vi "RTTrapTest-07-06-2017.vi"() -> ()   [LabVIEW 2010]
uses:
  <vilib>/userDefined/High Color/nirio_resource_hc.ctl
  <vilib>/rvi/interface/nirviOpenFPGA/nirviOpenFPGA.xnode
  C:/Users/HAGAR-IV/Desktop/Zeugs/markus/version feb 2012/FPGA Bitfiles/pertrasgcfpga2_FPGATarget_Trap1-06-06-2017_7789B2A8.lvbitx
  C:/Users/HAGAR-IV/Desktop/Zeugs/Johnny/pertrasgc fpga/Trap1-06-06-2017.vi
  <vilib>/rvi/ClientSDK/nirviWhatTheDeviceIsDoing.ctl
  <vilib>/rvi/interface/nirviReadWriteControl/nirviReadWriteControl.xnode
  <vilib>/rvi/interface/common/niFpgaNodeNameForErrorReporting.ctl
  <vilib>/rvi/errors/niLvFpgaWhatHappensToTopLevelVI.ctl
  <vilib>/rvi/interface/nirviMethod/nirviMethod.xnode
  <vilib>/rvi/interface/nirviCloseFPGA/nirviCloseFPGA.xnode
  <vilib>/FPGAPlugInAG/cRIO-9114/niLvFpga_Open_cRIO-9114.vi
  <vilib>/Utility/error.llb/Error Cluster From Error Code.vi
  <vilib>/rvi/errors/niLvFpgaAdjustHostInterfaceError.vi
  <vilib>/FPGAPlugInAG/cRIO-9114/niLvFpga_Close_cRIO-9114.vi
  NiFpgaLv.dll
panel:
  out "error out":errorcluster
  in  "Path":path=path "C:/TrapTest/Hotspot.txt"
  in  "Speichern":bool
  in  "Heizen-Ende":dbl=100.0
  out "PTStirling":dbl[](graph)
  in  "d1":fxp<+/-,21,21>=65000.0
  in  "d0 (100%=90000)":fxp<+/-,18,18>=6500.0
  in  "Vorlaufzeit":dbl=3.0
  in  "Heizung aus":bool
  out "Uhr":dbl
  in  "Heizen&Starten":bool
  in  "Rampenende":dbl
  in  "T2":dbl=50.0
  in  "T1":dbl=50.0
  out "ThermoTemp":dbl
  out "PTTempTrap":dbl[](graph)
  in  "ThermoKoeff0":dbl=12.98
  in  "ThermoKoeff2":dbl=-136.78
  in  "ThermoKoeff1":dbl=1284.53
  in  "PTStirlingKoeff0":dbl=-248.3
  in  "PTStirlingKoeff2":dbl=2.42
  in  "PTStirlingKoeff1":dbl=108.05
  in  "SollwertTemp":dbl=50.0
  in  "R(T)Koeff0":dbl=7.5948
  in  "R(T)Koeff2":dbl=6.486e-05
  in  "R(T)Koeff1":dbl=0.03631
  out "TempTrap":dbl[](graph)
  in  "Löschen":bool
  out "SollwertSchpannung":dbl
  out "SollwertWidrschtond":dbl=8.43
  out "TempTrap":dbl
  in  "T(R)Koeff0":dbl=-211.78
  in  "T(R)Koeff2":dbl=-0.47685
  in  "T(R)Koeff1":dbl=31.893
  out "WiderstandHeizdraht":dbl
  out "PTStirling":dbl format="%.2f"
  in  "Stirling":bool
  out "Thermo [V]":fxp<+/-,26,5> format="%.23g"
  in  "Heizen":bool
  out "Messwert":fxp<+/-,26,5> format="%.23g"
  in  "Warten(us)":u16=5000
  in  "stop":bool
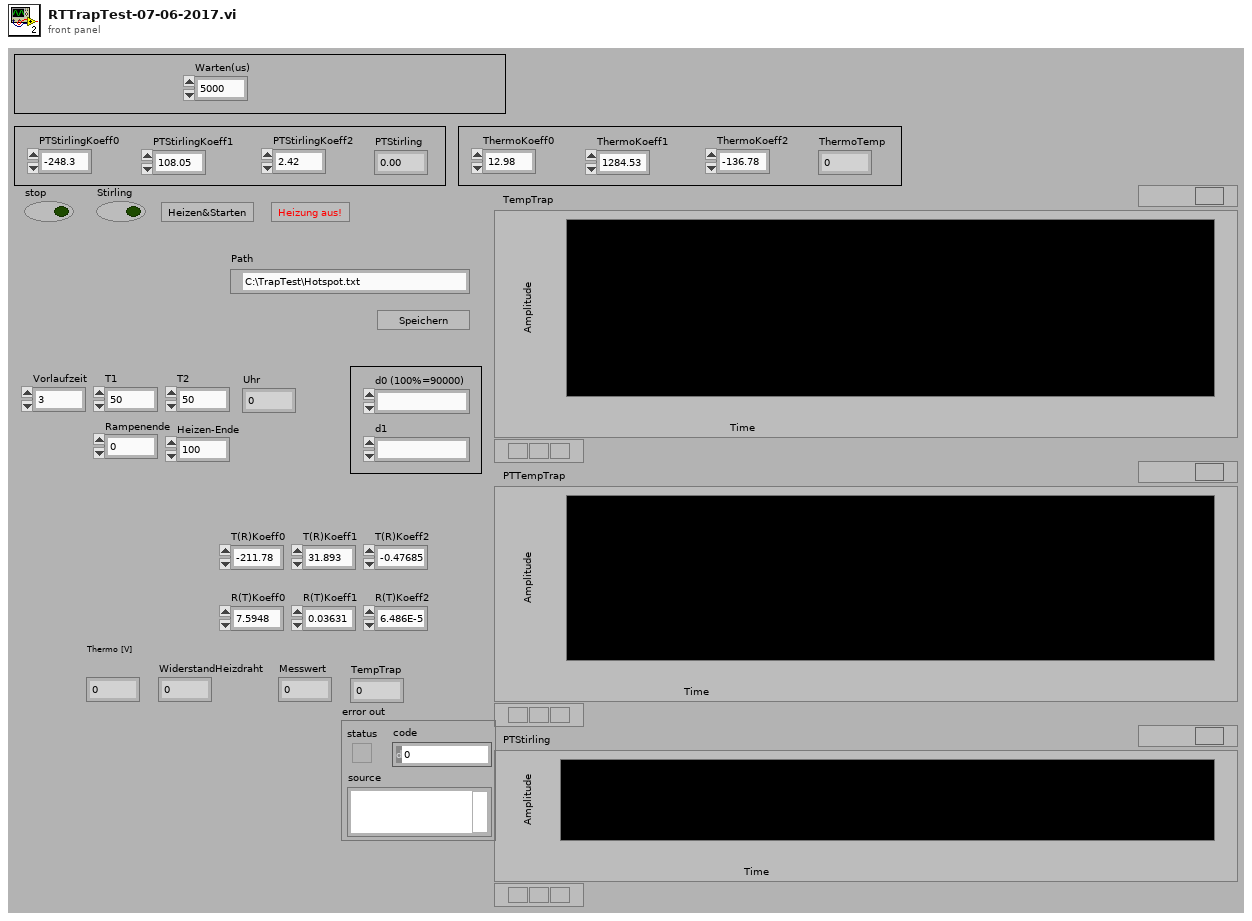
[diagram p1: front panel]
types:
  T1 = typedef "niFpgaNodeNameForErrorReporting.ctl" = enum16{"Open FPGA VI Reference", "Read/Write Control", "Invoke Method: Abort", "Invoke Method: Acknowledge IRQ", "Invoke Method: Download", "Invoke Method: FIFO.Configure", "Invoke Method: FIFO.Read", "Invoke Method: FIFO.Start", "Invoke Method: FIFO.Stop", "Invoke Method: FIFO.Write", "Invoke Method: Reset", "Invoke Method: Run", "Invoke Method: Wait on IRQ", "Close FPGA VI Reference"}
  T2 = typedef "niLvFpgaWhatHappensToTopLevelVI.ctl" = enum16{"top level VI scripted behind XNode", "top level VI inlined behind XNode"}
  T3 = enum16{"open", "replace", "create", "open or create", "replace or create", "replace or create with confirmation"}
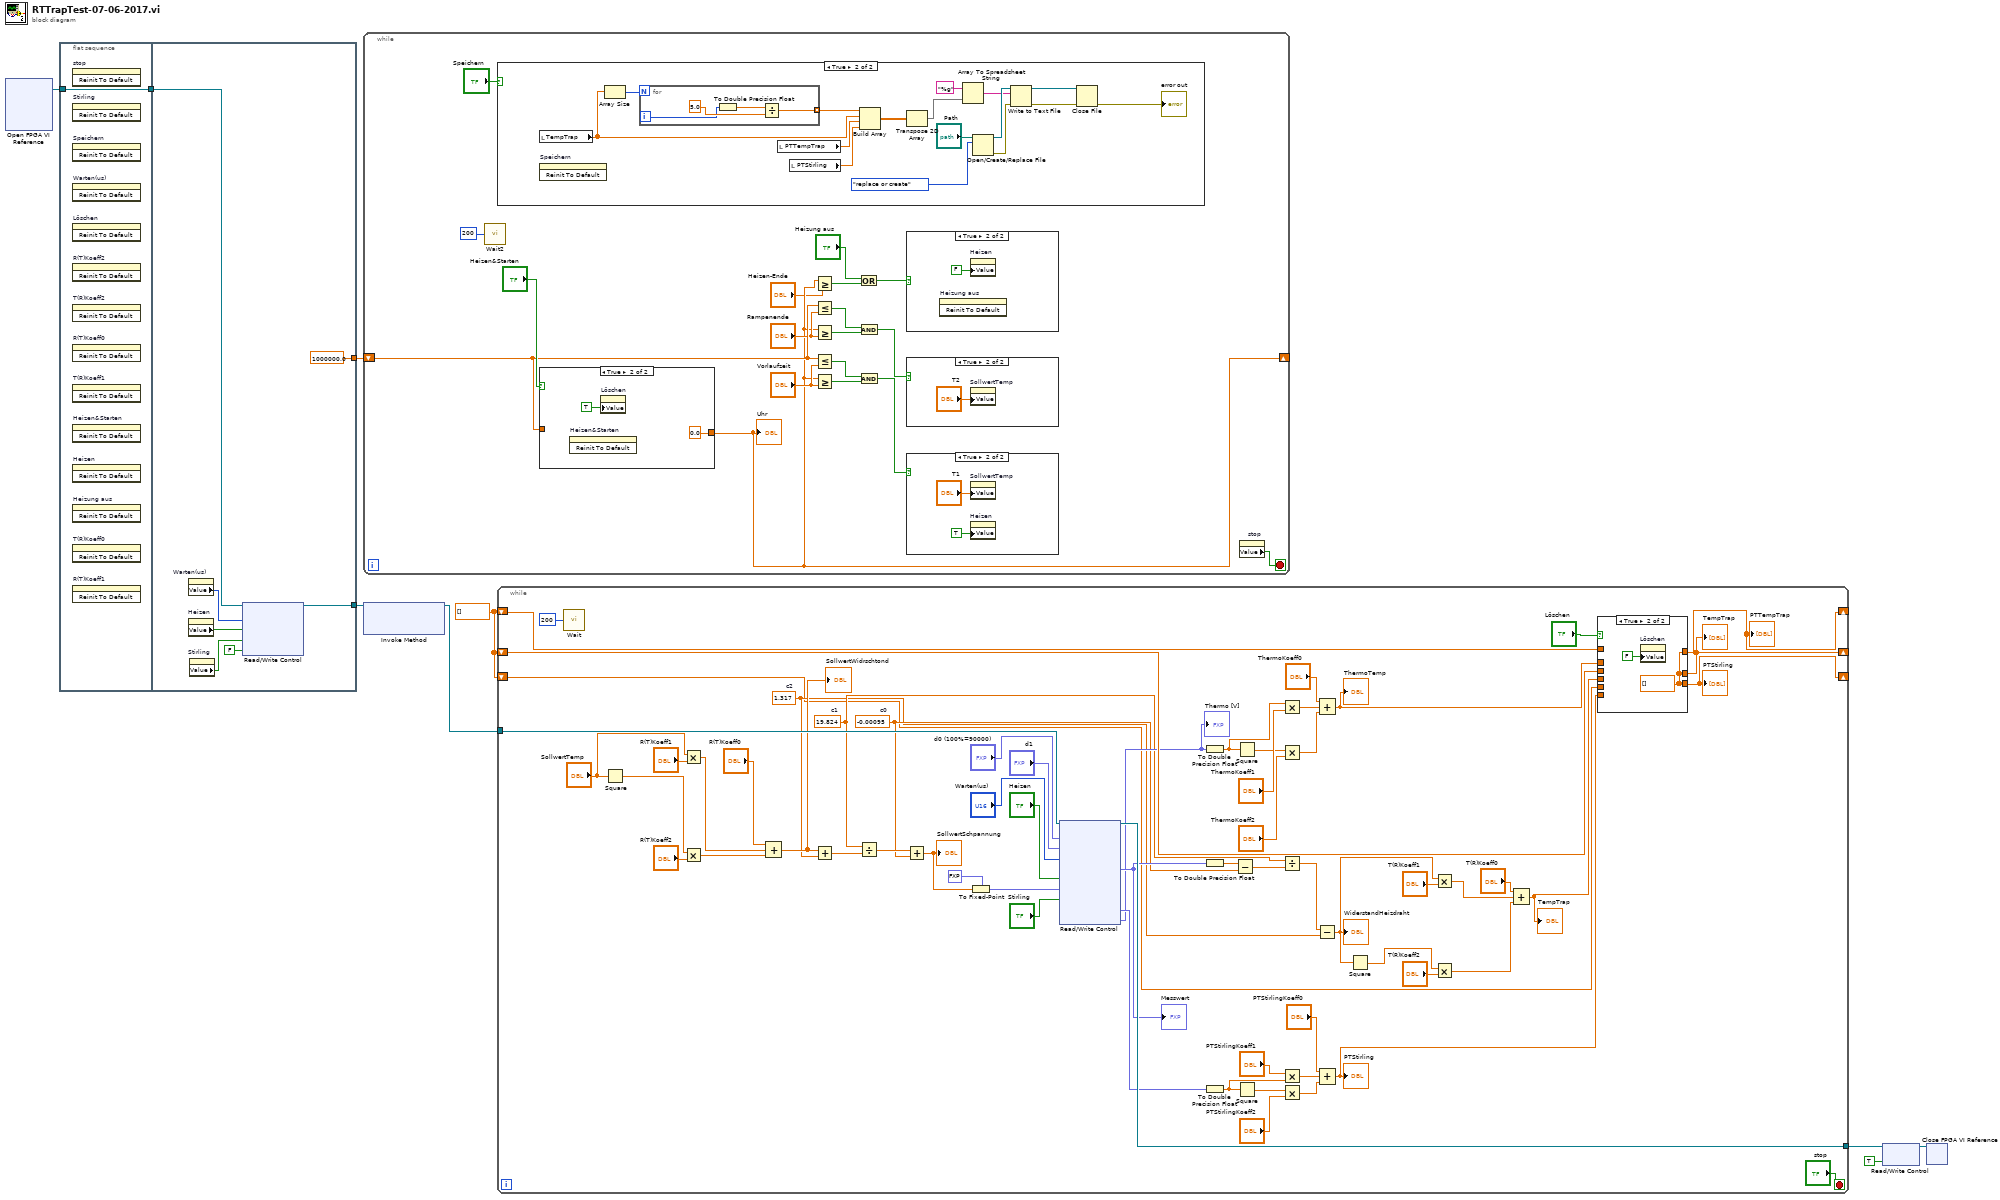
[diagram p0: block diagram]
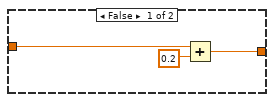
[diagram p6: hidden frame]
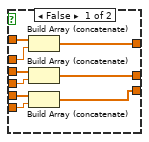
[diagram p7: hidden frame]
diagram:
  w1 = dbl[] []
  n1 = xnode "Open FPGA VI Reference"() -> ("FPGA VI Reference Out"=w9:refnum<k20>)  [unwired: 2 in, 1 out]
  n2 = flat-sequence {
    tunnel: w9 -> [w10]
    tunnel: [w10] -> w3
    tunnel: [w16] -> w8
    tunnel: w3 -> [w17]
    tunnel: [1000000.0] -> w2
    frame #0 {
      n3 = invoke on="stop" class="Bool (strict)" method="Reinit To Default"() -> ()  [unwired: 3 in, 3 out]
      n4 = invoke on="Stirling" class="Bool (strict)" method="Reinit To Default"() -> ()  [unwired: 3 in, 3 out]
      n5 = invoke on="Speichern" class="Bool" method="Reinit To Default"() -> ()  [unwired: 3 in, 3 out]
      n6 = invoke on="Warten(us)" class="DigNum (strict)" method="Reinit To Default"() -> ()  [unwired: 3 in, 3 out]
      n7 = invoke on="Löschen" class="Bool (strict)" method="Reinit To Default"() -> ()  [unwired: 3 in, 3 out]
      n8 = invoke on="R(T)Koeff2" class="DigNum (strict)" method="Reinit To Default"() -> ()  [unwired: 3 in, 3 out]
      n9 = invoke on="T(R)Koeff2" class="DigNum (strict)" method="Reinit To Default"() -> ()  [unwired: 3 in, 3 out]
      n10 = invoke on="R(T)Koeff0" class="DigNum (strict)" method="Reinit To Default"() -> ()  [unwired: 3 in, 3 out]
      n11 = invoke on="T(R)Koeff1" class="DigNum (strict)" method="Reinit To Default"() -> ()  [unwired: 3 in, 3 out]
      n12 = invoke on="Heizen&Starten" class="Bool" method="Reinit To Default"() -> ()  [unwired: 3 in, 3 out]
      n13 = invoke on="Heizen" class="Bool (strict)" method="Reinit To Default"() -> ()  [unwired: 3 in, 3 out]
      n14 = invoke on="Heizung aus" class="Bool" method="Reinit To Default"() -> ()  [unwired: 3 in, 3 out]
      n15 = invoke on="T(R)Koeff0" class="DigNum (strict)" method="Reinit To Default"() -> ()  [unwired: 3 in, 3 out]
      n16 = invoke on="R(T)Koeff1" class="DigNum (strict)" method="Reinit To Default"() -> ()  [unwired: 3 in, 3 out]
    }
    frame #1 {
      n17 = property on="Warten(us)" class="DigNum (strict)"() -> ("Value"=w15:u16)  [unwired: 2 in, 2 out]
      n18 = property on="Heizen" class="Bool (strict)"() -> ("Value"=w14:bool)  [unwired: 2 in, 2 out]
      n19 = property on="Stirling" class="Bool (strict)"() -> ("Value"=w13:bool)  [unwired: 2 in, 2 out]
      n20 = xnode "Read/Write Control"("FPGA VI Reference In"=w17, "Warten(uSec)"=w15, "heizen"=w14, "Stirling"=w13, "stop"=FALSE) -> ("FPGA VI Reference Out"=w16:refnum<k20>)  [unwired: 1 in, 1 out]
    }
  }
  n21 = while {
    shift-right: [w119] -> _
    shift-left: w2 -> [w128]
    stop <- w134 stop-if-true
    n22 = call "Wait2"("Count(mSec)"=u32 200) -> ()  [unwired: 1 out]
    n23 = case shown="True" "Speichern" {
      frame False {
      }
      frame True {
        n24 = local read "TempTrap"() -> (w138:dbl[])
        n25 = invoke on="Speichern" class="Bool" method="Reinit To Default"() -> ()  [unwired: 3 in, 3 out]
        n26 = Array Size(array=w138) -> (size(s)=w137:i32)
        n27 = for {
          N: w137 -> [_]
          tunnel: [w153] -> w136 mode=indexing
          i -> [w152]
          n28 = To Double Precision Float(number=w152) -> (double precision float=w154:dbl)
          n29 = Divide(x=w154, y=5.0) -> (x/y=w153:dbl)
        }
        n30 = local read "PTTempTrap"() -> (w142:dbl[])
        n31 = local read "PTStirling"() -> (w141:dbl[])
        n32 = Build Array(w136, w138, w142, w141) -> (w140:dbl[][])
        n33 = Transpose 2D Array(2D array=w140) -> (transposed array=w139:dbl[][])
        n34 = Array To Spreadsheet String(array=w139, 3:"%g" ("format string")) -> (spreadsheet string=w143:string)  [unwired: 1 in]
        n35 = Open/Create/Replace File(file path (use dialog)="Path", operation (0:open)=T3."replace or create") -> (refnum out=w149:refnum<file>, error out=w148:errorcluster)  [unwired: 4 in, 1 out]
        n36 = Write to Text File(file (use dialog)=w149, text=w143, error in=w148) -> (refnum out=w147:refnum<file>, error out=w146:errorcluster)  [unwired: 1 in, 1 out]
        n37 = Close File(refnum=w147, error in=w146) -> (error out=→"error out":errorcluster)  [unwired: 1 out]
      }
    }
    n38 = case shown="True" "Heizen&Starten" {
      tunnel: w128 -> [w162 _]
      tunnel: [w160 0.0 ("t")] -> w119
      frame False {
        n39 = Add(x=w162, y=0.2) -> (x+y=w160:dbl)
      }
      frame True {
        n40 = invoke on="Heizen&Starten" class="Bool" method="Reinit To Default"() -> ()  [unwired: 3 in, 3 out]
        n41 = property on="Löschen" class="Bool (strict)"("Value"=TRUE ("Löschen")) -> ()  [unwired: 2 in, 2 out]
      }
    }
    "Uhr" <- w119
    n42 = Greater Or Equal?(x=w119, y="Heizen-Ende") -> (x >= y?=w122:bool)
    n43 = Less Or Equal?(x=w128, y="Rampenende") -> (x <= y?=w126:bool)
    n44 = Greater Or Equal?(x=w119, y="Rampenende") -> (x >= y?=w125:bool)
    n45 = Less Or Equal?(x=w128, y="Vorlaufzeit") -> (x <= y?=w130:bool)
    n46 = Greater Or Equal?(x=w119, y="Vorlaufzeit") -> (x >= y?=w131:bool)
    n47 = Or(x="Heizung aus", y=w122) -> (x .or. y?=w121:bool)
    n48 = And(x=w126, y=w125) -> (x .and. y?=w124:bool)
    n49 = And(x=w130, y=w131) -> (x .and. y?=w129:bool)
    n50 = case shown="True" w121 {
      frame False {
      }
      frame True {
        n51 = invoke on="Heizung aus" class="Bool" method="Reinit To Default"() -> ()  [unwired: 3 in, 3 out]
        n52 = property on="Heizen" class="Bool (strict)"("Value"=FALSE ("Heizen")) -> ()  [unwired: 2 in, 2 out]
      }
    }
    n53 = case shown="True" w124 {
      frame False {
      }
      frame True {
        n54 = property on="SollwertTemp" class="DigNum (strict)"("Value"="T2") -> ()  [unwired: 2 in, 2 out]
      }
    }
    n55 = case shown="True" w129 {
      frame False {
      }
      frame True {
        n56 = property on="SollwertTemp" class="DigNum (strict)"("Value"="T1") -> ()  [unwired: 2 in, 2 out]
        n57 = property on="Heizen" class="Bool (strict)"("Value"=TRUE ("Heizen")) -> ()  [unwired: 2 in, 2 out]
      }
    }
    n58 = property on="stop" class="Bool (strict)"() -> ("Value"=w134:bool)  [unwired: 2 in, 2 out]
  }
  n59 = xnode "Invoke Method"("FPGA VI Reference In"=w8) -> ("FPGA VI Reference Out"=w7:refnum<k20>)  [unwired: 2 in, 1 out]
  n60 = while {
    tunnel: w7 -> [w226]
    tunnel: [w224] -> w6
    shift-right: [w207] -> _
    shift-left: w1 -> [w209]
    shift-right: [w182] -> _
    shift-left: w1 -> [w191]
    shift-right: [w165] -> _
    shift-left: w1 -> [w167]
    stop <- "stop" stop-if-true
    w169 = 1.317  # c2
    w172 = 19.824  # c1
    w173 = -0.00095  # c0
    n61 = call "Wait"("Count(mSec)"=u32 200) -> ()  [unwired: 1 out]
    n62 = Square(x="SollwertTemp") -> (x^2=w206:dbl)
    n63 = Multiply(x="SollwertTemp", y="R(T)Koeff1") -> (x*y=w201:dbl)
    n64 = Multiply(x=w206, y="R(T)Koeff2") -> (x*y=w200:dbl)
    n65 = Compound Arithmetic op=ADD("R(T)Koeff0", w201, w200) -> (w178:dbl)
    "SollwertWidrschtond" <- w178
    n66 = Add(x=w178, y=w169) -> (x+y=w177:dbl)
    n67 = Divide(x=w172, y=w177) -> (x/y=w176:dbl)
    n68 = Add(x=w176, y=w173) -> (x+y=w175:dbl)
    "SollwertSchpannung" <- w175
    n69 = To Fixed-Point(fixed-point type=fxp<+/-,26,5> 0.0 ("setpoint"), number=w175) -> (fixed-point=w212:fxp<+/-,26,5>)
    n70 = xnode "Read/Write Control"("FPGA VI Reference In"=w226, "d0"="d0 (100%=90000)", "d1"="d1", "Warten(uSec)"="Warten(us)", "heizen"="Heizen", "U_SP"=w212, "Stirling"="Stirling") -> ("FPGA VI Reference Out"=w224:refnum<k20>, "U_MW"=w214:fxp<+/-,26,5>, "PTStirling"=w192:fxp<+/-,26,5>, "PreCol1_MW"=w181:fxp<+/-,26,5>)  [unwired: 1 in, 1 out]
    "Messwert" <- w214
    "Thermo [V]" <- w181
    n71 = To Double Precision Float(number=w181) -> (double precision float=w187:dbl)
    n72 = To Double Precision Float(number=w214) -> (double precision float=w174:dbl)
    n73 = To Double Precision Float(number=w192) -> (double precision float=w198:dbl)
    n74 = Subtract(x=w174, y=w173) -> (x-y=w171:dbl)
    n75 = Square(x=w187) -> (x^2=w186:dbl)
    n76 = Square(x=w198) -> (x^2=w197:dbl)
    n77 = Multiply(x=w187, y="ThermoKoeff1") -> (x*y=w188:dbl)
    n78 = Multiply(x=w186, y="ThermoKoeff2") -> (x*y=w184:dbl)
    n79 = Divide(x=w172, y=w171) -> (x/y=w170:dbl)
    n80 = Multiply(x="PTStirlingKoeff1", y=w198) -> (x*y=w194:dbl)
    n81 = Multiply(x=w197, y="PTStirlingKoeff2") -> (x*y=w193:dbl)
    n82 = Subtract(x=w170, y=w169) -> (x-y=w168:dbl)
    "WiderstandHeizdraht" <- w168
    n83 = Compound Arithmetic op=ADD("ThermoKoeff0", w188, w184) -> (w183:dbl)
    "ThermoTemp" <- w183
    n84 = Compound Arithmetic op=ADD("PTStirlingKoeff0", w194, w193) -> (w166:dbl)
    "PTStirling" <- w166
    n85 = Square(x=w168) -> (x^2=w219:dbl)
    n86 = Multiply(x=w168, y="T(R)Koeff1") -> (x*y=w216:dbl)
    n87 = Multiply(x=w219, y="T(R)Koeff2") -> (x*y=w217:dbl)
    n88 = Compound Arithmetic op=ADD("T(R)Koeff0", w216, w217) -> (w210:dbl)
    "TempTrap" <- w210
    n89 = case shown="True" "Löschen" {
      tunnel: w210 -> [w235 _]
      tunnel: [w234 w236] -> w207
      tunnel: w209 -> [w233 _]
      tunnel: [w232 w236] -> w182
      tunnel: w191 -> [w231 _]
      tunnel: w183 -> [w230 _]
      tunnel: [w229 w236] -> w165
      tunnel: w167 -> [w228 _]
      tunnel: w166 -> [w227 _]
      frame False {
        n90 = Build Array (concatenate)(w231, w230) -> (w232:dbl[])
        n91 = Build Array (concatenate)(w233, w235) -> (w234:dbl[])
        n92 = Build Array (concatenate)(w228, w227) -> (w229:dbl[])
      }
      frame True {
        w236 = dbl[] []
        n93 = property on="Löschen" class="Bool (strict)"("Value"=FALSE ("Löschen")) -> ()  [unwired: 2 in, 2 out]
      }
    }
    "TempTrap" <- w207
    "PTTempTrap" <- w182
    "PTStirling" <- w165
  }
  n94 = xnode "Read/Write Control"("FPGA VI Reference In"=w6, "stop"=TRUE) -> ("FPGA VI Reference Out"=w4:refnum<k20>)  [unwired: 1 in, 1 out]
  n95 = xnode "Close FPGA VI Reference"("FPGA VI Reference In"=w4) -> ()  [unwired: 1 in, 1 out]
